vi "Compuerta_Sat.vi"(4 "BCHECK":bool, 6 "FALLA UU":bool, 8 "FALLA CD":bool, 9 "FALLA CU":bool, 10 "CONSOLIDACION":bool, 11 "SATURACION":bool) -> (3 "Boolean":bool)   [LabVIEW 2015]
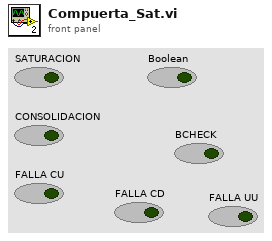
[diagram p1: front panel]
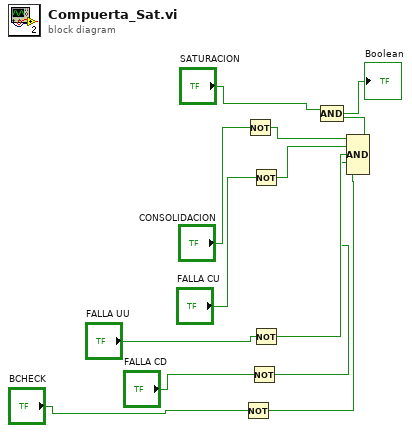
[diagram p0: block diagram]
diagram:
  n1 = Not(x="BCHECK") -> (.not. x?=w4:bool)
  n2 = Not(x="CONSOLIDACION") -> (.not. x?=w8:bool)
  n3 = Not(x="FALLA CD") -> (.not. x?=w5:bool)
  n4 = Not(x="FALLA CU") -> (.not. x?=w7:bool)
  n5 = Not(x="FALLA UU") -> (.not. x?=w6:bool)
  n6 = Compound Arithmetic op=AND(w8, w7, w6, w5, w4) -> (w10:bool)
  n7 = Compound Arithmetic op=AND("SATURACION", w10) -> (→"Boolean":bool)
